vi "GetParam.vi"(8 "error in (no error)":errorcluster caption="entrée d'erreur (pas d'erreur)", 11 "Fowlkes_Mallows_Score.lvclass":refnum<class "Fowlkes_Mallows_Score.lvclass">) -> (0 "error out":errorcluster caption="sortie d'erreur", 2 "fowlkes_mallows_score":cluster{"sparse":bool}, 3 "Fowlkes_Mallows_Score.lvclass":refnum<class "Fowlkes_Mallows_Score.lvclass">)   [LabVIEW 2020, in "Fowlkes_Mallows_Score.lvclass"]
doc: "Get Parameters"
uses:
  Fowlkes_Mallows_Score.lvclass
  Fowlkes_Mallows_Score.lvclass/Fowlkes_Mallows_Score.ctl
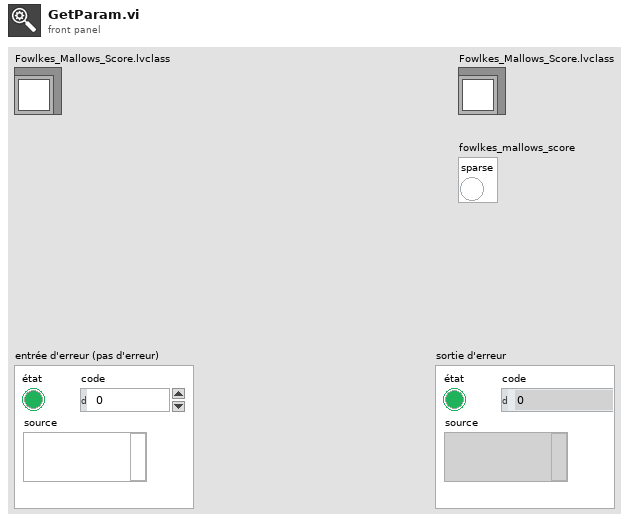
[diagram p1: front panel]
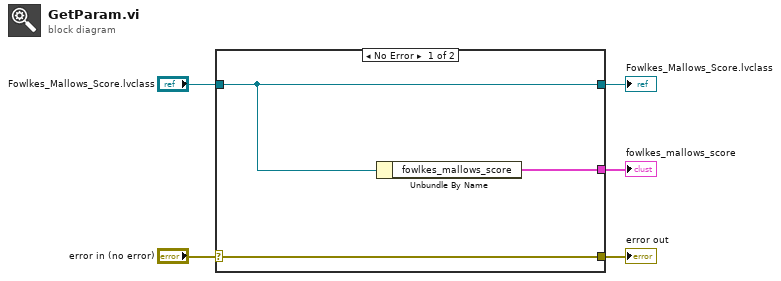
[diagram p0: block diagram]
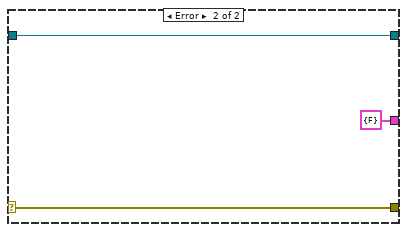
[diagram p2: hidden frame]
diagram:
  n1 = case shown="No Error" "error in (no error)" {
    selector: "error in (no error)" -> [w8 w10]
    tunnel: [w8 w10] -> w4
    tunnel: [w7 w11] -> w2
    tunnel: "Fowlkes_Mallows_Score.lvclass" -> [w7 w11]
    tunnel: [w6 cluster{"sparse":bool} {"sparse"=FALSE} ("fowlkes_mallows_score")] -> w1
    frame No Error {
      n2 = Unbundle By Name(w7) -> ("fowlkes_mallows_score"=w6:cluster{"sparse":bool})
    }
    frame Error {
    }
  }
  "error out" <- w4
  "Fowlkes_Mallows_Score.lvclass" <- w2
  "fowlkes_mallows_score" <- w1
